vi "Prober_CloseSession.vi"(8 "error in (no error)":errorcluster, 11 "AlessiRel6100 in":refnum<class "AlessiRel6100.lvclass">) -> (0 "error out":errorcluster, 3 "AlessiRel6100 out":refnum<class "AlessiRel6100.lvclass">)   [LabVIEW 2018, in "AlessiRel6100.lvclass"]
uses:
  AlessiRel6100.lvclass
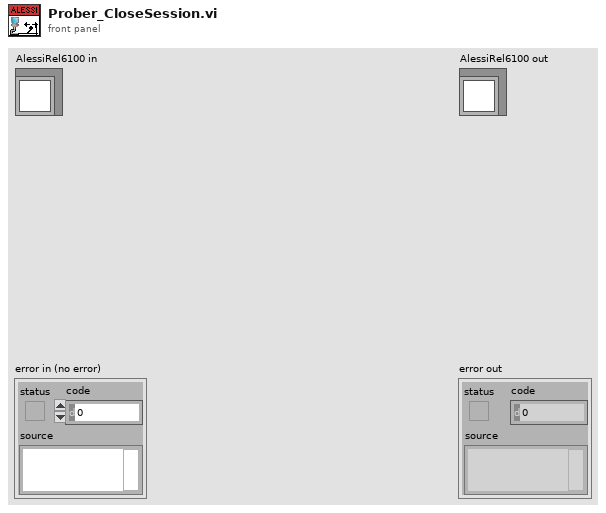
[diagram p1: front panel]
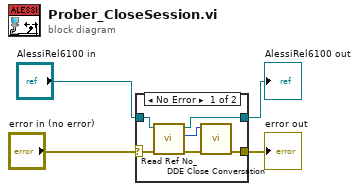
[diagram p0: block diagram]
diagram:
  n1 = case shown="No Error" "error in (no error)" {
    selector: "error in (no error)" -> [w9 w11]
    tunnel: "AlessiRel6100 in" -> [w10 w12]
    tunnel: [w7 w11] -> w2
    tunnel: [w5 w12] -> w1
    frame No Error {
      n2 = call-dynamic "Read Ref No_.vi"("error in (no error)"=w9, "AlessiRel6100 in"=w10) -> ("error out"=w8:errorcluster, "Ref No."=w6:u32, "AlessiRel6100 out"=w5:refnum<class "AlessiRel6100.lvclass">)  [unwired: 7 in]
      n3 = call "DDE Close Conversation.vi"("error in (no error)"=w8, "conversation refnum"=w6) -> ("error out"=w7:errorcluster)  [unwired: 7 in]
    }
    frame Error {
    }
  }
  "error out" <- w2
  "AlessiRel6100 out" <- w1
